vi "Strongrid_Core_app.vi"() -> ()   [LabVIEW 2013]
uses:
  Dependencies/Freq_select.ctl
  Dependencies/FrequencyKnob.ctl
  <vilib>/lvdsc/process/Undeploy Library.vi
  <vilib>/lvdsc/process/Deploy Library.vi
  <vilib>/S3DK/PMU Recorder Light/PMU Recorder Light.lvlib
  <vilib>/lvdsc/NI_DSC.lvlib
panel:
  in  "Ipad ON":bool
  in  "Ipad Display":bool
  out "low":bool caption="Low Frequency Warning"
  out "high":bool caption="High Frequency Warning"
  out "Xtra low":bool caption="Low Frequency Alarm"
  out "Xtra high":bool caption="High Frequency Alarm"
  out "TAMPERE":bool
  out "Aalto":bool
  out "Aalto Voltage":sgl
  out "Aalto Freq":T1 scale=49.85..50.15
  in  "V_select":T2 caption="Voltage Selection"
  out "Lund Frequency":T1 scale=49.85..50.15
  in  "Open PRL":bool
  out "Phasors":picture
  out "Buffer Active":bool
  out "Configuration File Received":bool
  out "Connected":bool
  out "Status Loop":bool
  out "Error":bool
  out "KTH Voltage":sgl
  out "KTH Frequency":T1 scale=49.85..50.15
  out "Chalmers Voltage":sgl
  out "Lund Voltage":sgl
  out "Tampere Voltage":sgl
  out "NTNU Voltage":sgl
  out "Tampere Frequency":T1 scale=49.85..50.15
  out "Chalmers Frequency":T1 scale=49.85..50.15
  out "NTNU Frequency":T1 scale=49.85..50.15
  out "LTU Voltage":sgl
  out "LTU Freq":T1 scale=49.85..50.15
  out "Lund PMU":bool
  out "Chalmers PMU":bool
  out "KTH PMU":bool
  out "NTNU PMU":bool
  out "LTU PMU":bool
  out "Has New Data?":bool
  out "Timed Loop":bool
  in  "Get Full Buffer?":bool
  in  "f_select":T2 caption="Frequency Selection"
  in  "Refresh Rate":u32(ring)=200 items=["20 Hz"=50, "10 Hz"=100, "5 Hz"=200, "2 Hz"=500, "1 Hz"=1000, "Every 2 sec"=2000, "Every 5 sec"=5000, "Every 10 sec"=10000, "Every minute"=4294961760]
  out "Quitting":bool
  out "Execution Loop":bool
  in  "Quit":bool
  out "Event Loop":bool
  out "Frequency":waveform(sgl)[](graph)
  out "Voltage":waveform(sgl)[](graph)
  # "USAGE:  Press play. The VI will start the PRL itself and wait for the connection to be established.\n(you will still need to configure the PRL first. If the Simple Frequency Reader works, then this works)"
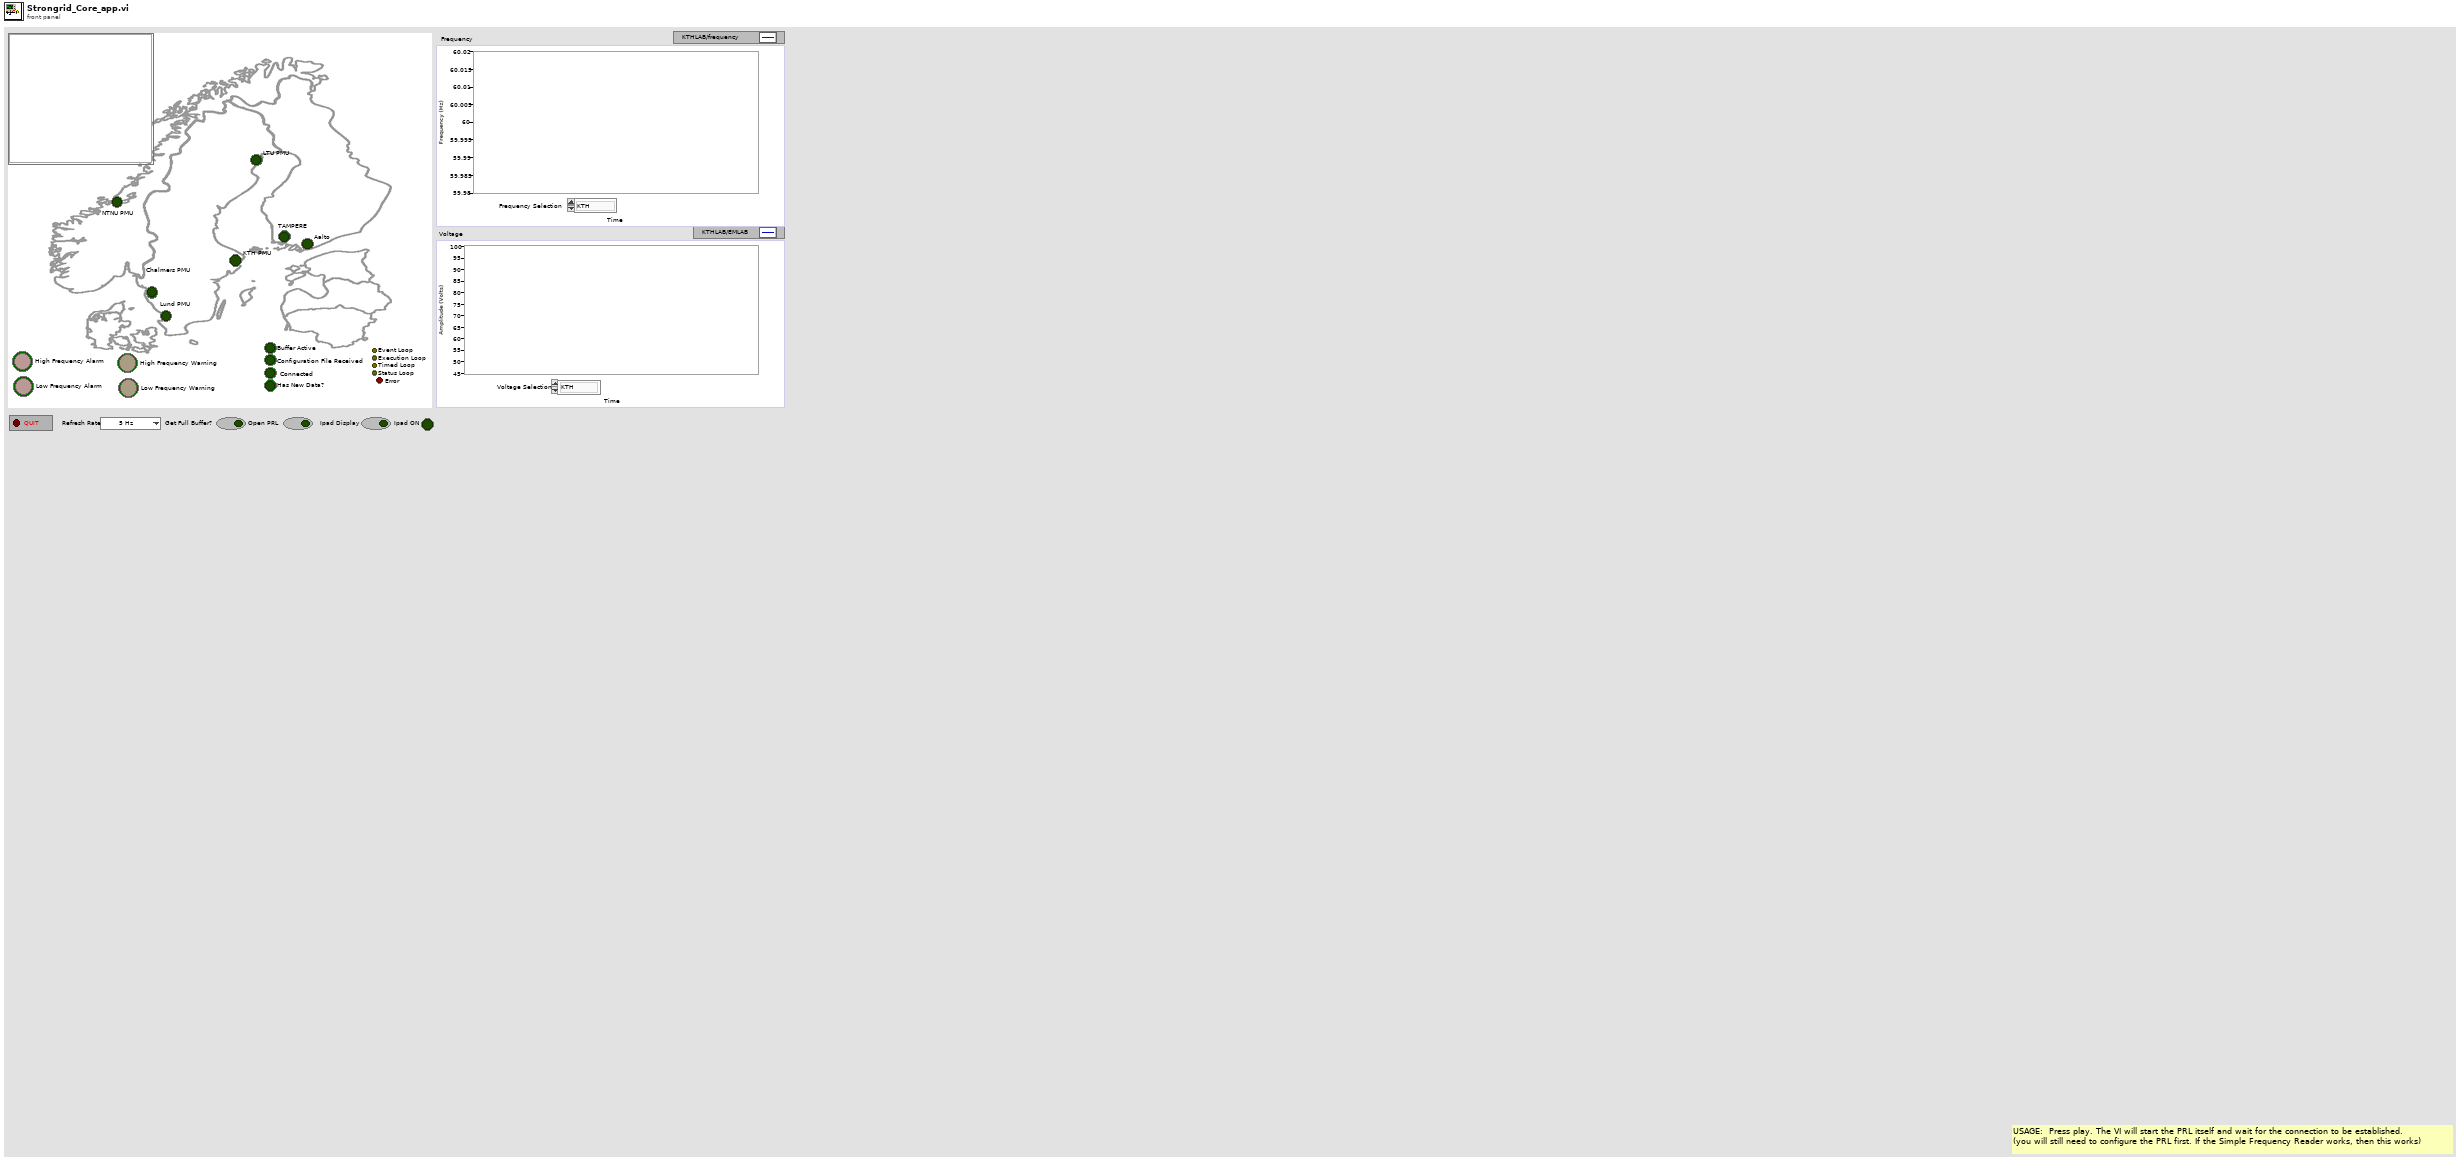
[diagram p1: front panel]
types:
  T1 = typedef "FrequencyKnob.ctl" = sgl
  T2 = typedef "Freq_select.ctl" = enum16{"KTH", "NTNU", "LTH", "CTH", "TAMPERE", "LTU", "Aalto", "ALL"}
  T3 = typedef "Semaphore RefNum" = refnum<k1>
  T4 = typedef "LVBoundsTypeDef.ctl" = cluster{"Width":u32, "Height":u32}
  T5 = enum16{"Run", "Startup", "Get Status", "Pause", "Continue", "Shutdown", "Abort", "Open Panel", "Close Panel"}
  T6 = cluster{"Phasor":string[], "Analog":string[], "Digital":string[]}
  T7 = enum16{"Filter Signals", "Get All Signal Names", "Select Signals on Name", "Select Frequency Only", "Get Selected Signal Names"}
  T8 = cluster{"KTH Voltage":refnum<vi>, "KTH Frequency":refnum<vi>}
  T9 = cluster{"LTU Voltage":refnum<vi>, "LTU Freq":refnum<vi>}
  T10 = cluster{"NTNU Voltage":refnum<vi>, "NTNU Frequency":refnum<vi>}
  T11 = cluster{"Chalmers Voltage":refnum<vi>, "Chalmers Frequency":refnum<vi>}
  T12 = cluster{"Lund Voltage":refnum<vi>, "Lund Frequency":refnum<vi>}
  T13 = cluster{"Tampere Voltage ":refnum<vi>, "Tampere Frequency":refnum<vi>}
  T14 = cluster{"Aalto Voltage":refnum<vi>, "Aalto Freq":refnum<vi>}
  T15 = cluster{"Analog Signals[0]":sgl, "Analog Signals[1]":sgl, "Analog Signals[2]":sgl, "Analog Signals[3]":sgl, "Analog Signals[4]":sgl, "Analog Signals[5]":sgl, "Analog Signals[6]":sgl}
  T16 = cluster{"[0]":sgl, "[1]":sgl, "[2]":sgl, "[3]":sgl, "[4]":sgl, "[5]":sgl, "[6]":sgl}
  T17 = cluster{"[0]":bool, "[1]":bool, "[2]":bool, "[3]":bool, "[4]":bool, "[5]":bool, "[6]":bool}
  T18 = cluster{"KTH":sgl, "NTNU":sgl, "Lund":sgl, "Chalmers":sgl, "Tampere":sgl, "LTU":sgl, "Aalto":sgl}
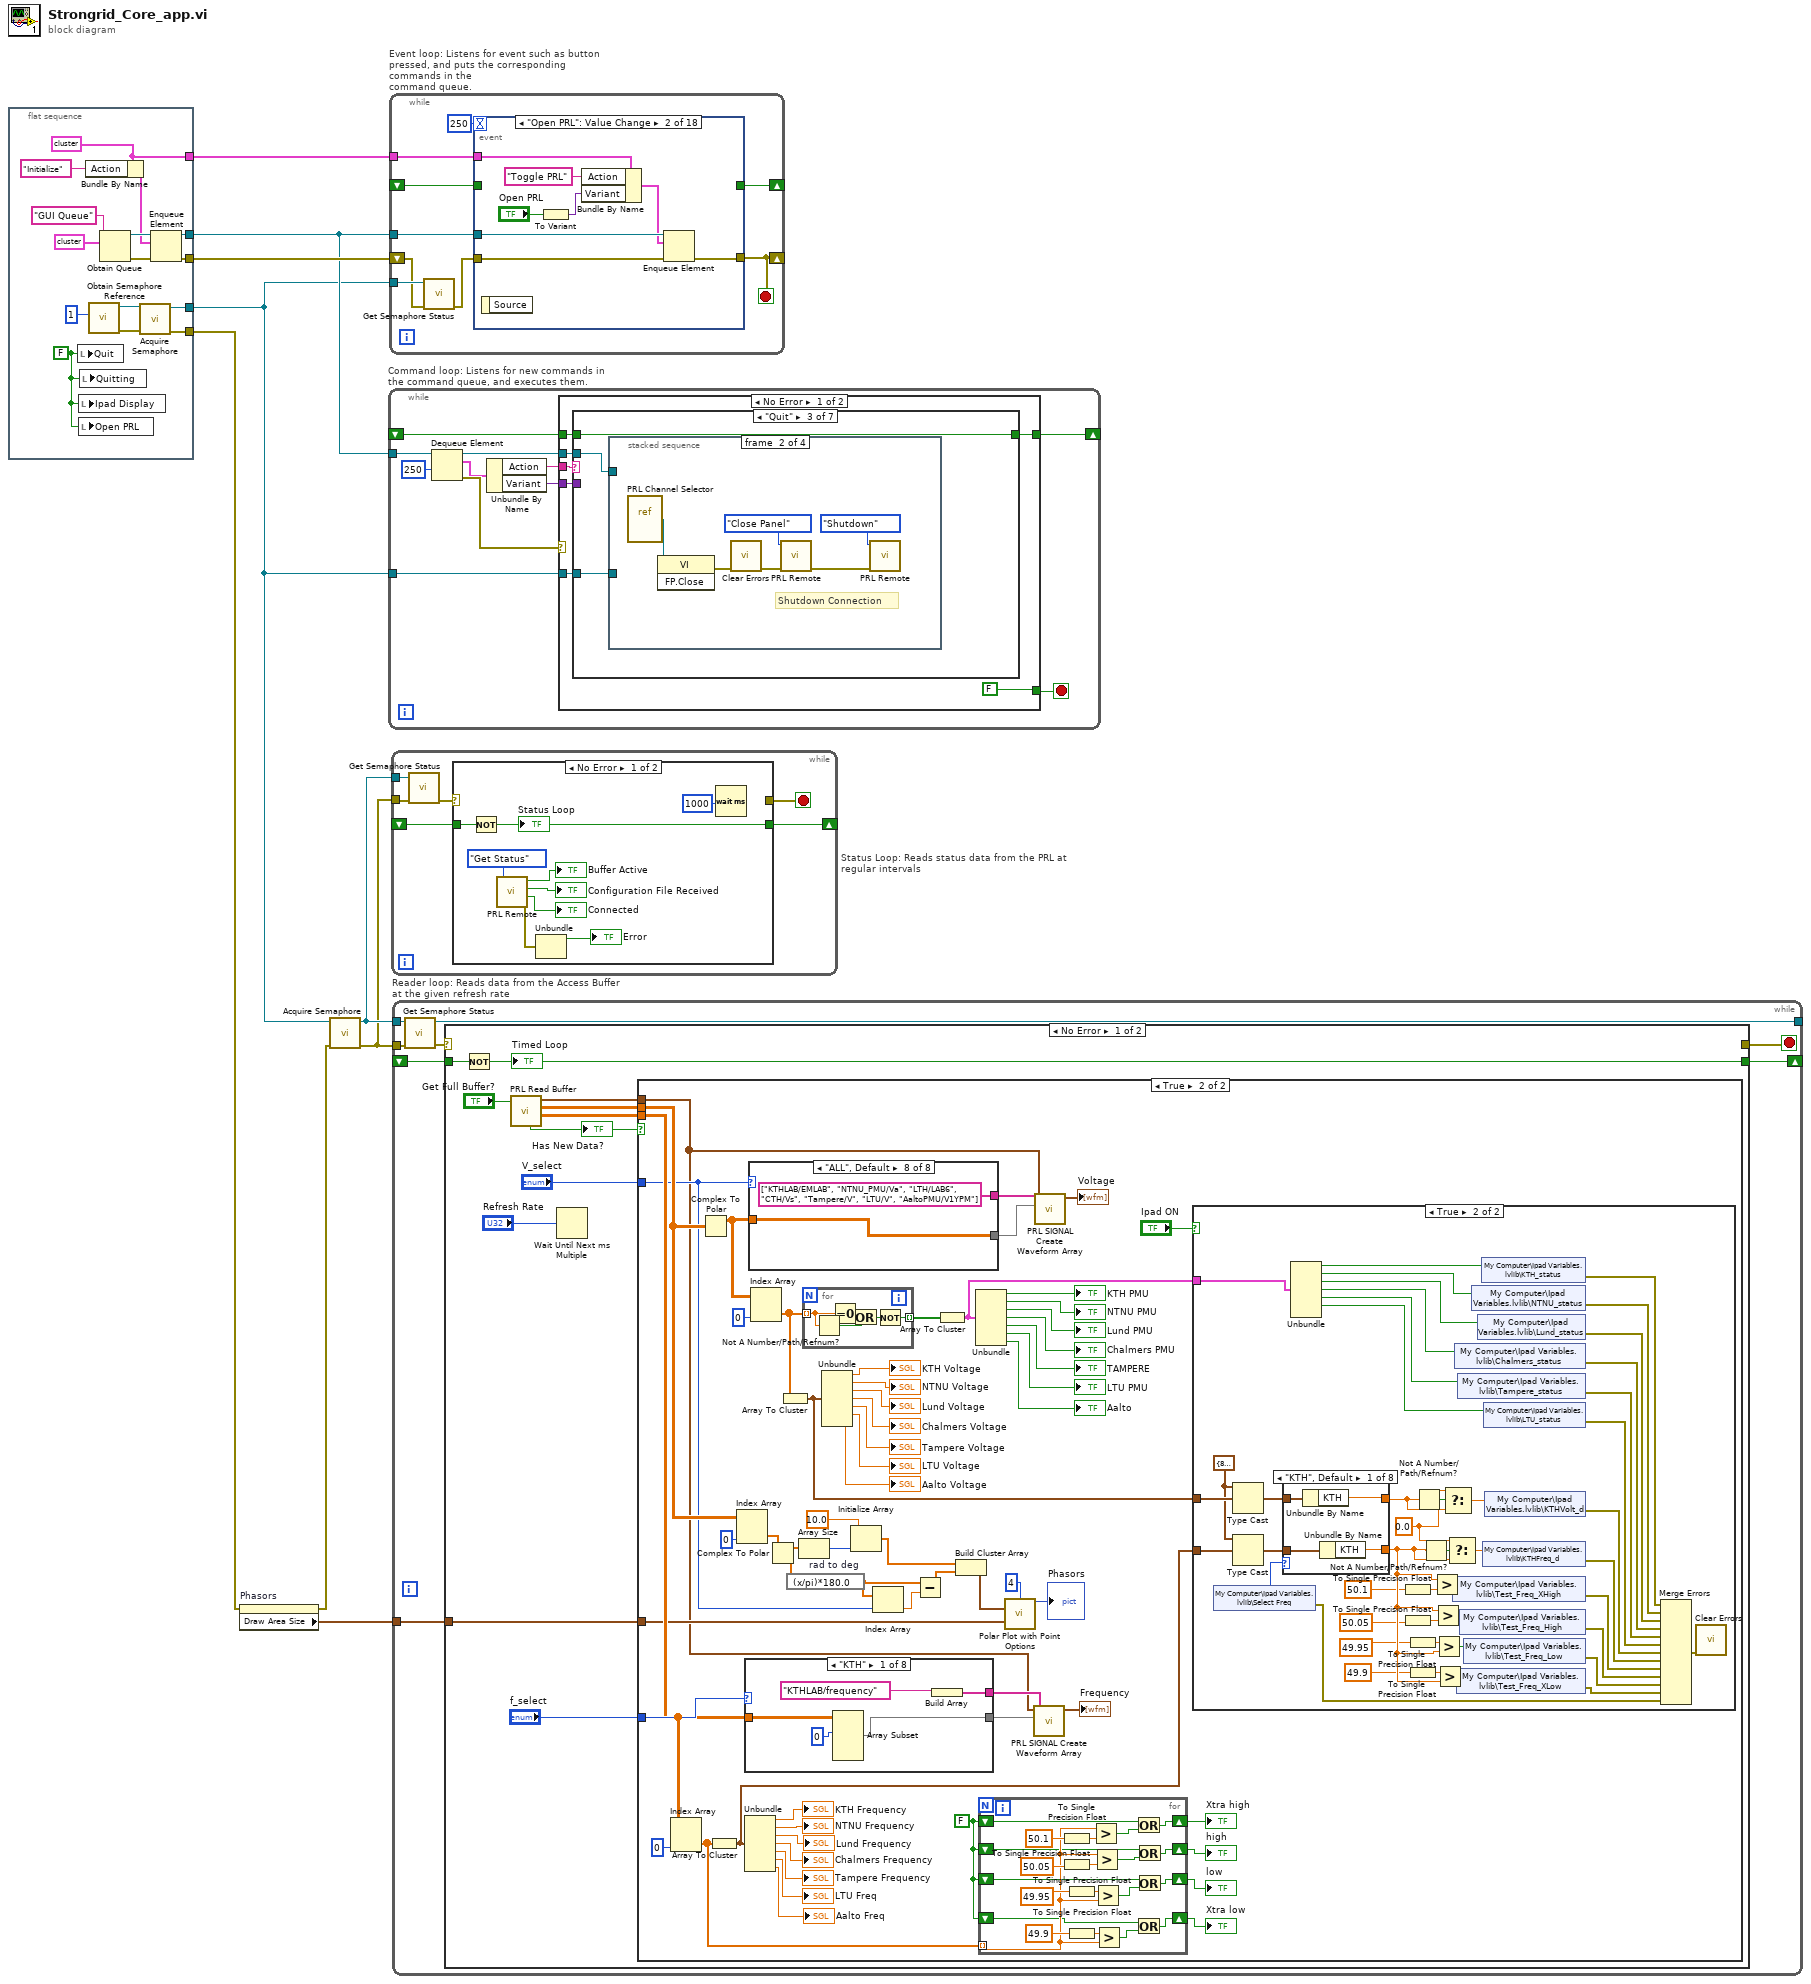
[diagram p0: block diagram]
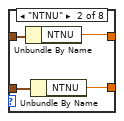
[diagram p5: hidden frame]
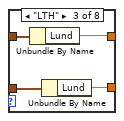
[diagram p6: hidden frame]
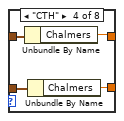
[diagram p7: hidden frame]
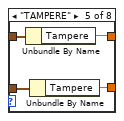
[diagram p8: hidden frame]
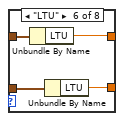
[diagram p9: hidden frame]
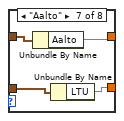
[diagram p10: hidden frame]
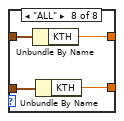
[diagram p11: hidden frame]
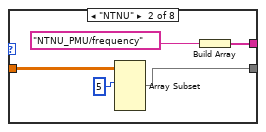
[diagram p12: hidden frame]
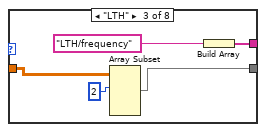
[diagram p13: hidden frame]
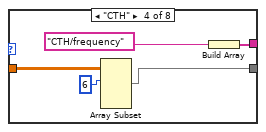
[diagram p14: hidden frame]
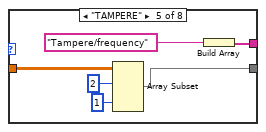
[diagram p15: hidden frame]
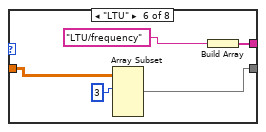
[diagram p16: hidden frame]
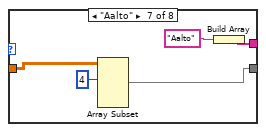
[diagram p17: hidden frame]
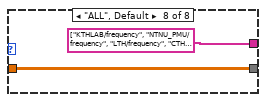
[diagram p18: hidden frame]
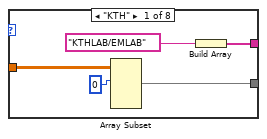
[diagram p19: hidden frame]
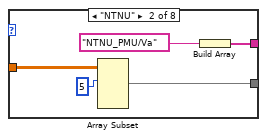
[diagram p20: hidden frame]
diagram:
  n1 = flat-sequence {
    tunnel: [w22] -> w9
    tunnel: [w21] -> w8
    tunnel: [w16] -> w7
    tunnel: [w12] -> w2
    tunnel: [w11] -> w1
    frame #0 {
      w10 = FALSE ("Quit")
      w16 = cluster{"Variant":variant, "Action":string} {"Variant"=variant, "Action"=""} ("Queue Element")
      n2 = local write "Quit"(w10) -> ()
      n3 = local write "Ipad Display"(w10) -> ()
      n4 = local write "Open PRL"(w10) -> ()
      n5 = local write "Quitting"(w10) -> ()
      n6 = Bundle By Name(cluster=w16, "Action"="Initialize" ("element")) -> (w17:cluster{"Variant":variant, "Action":string})
      n7 = call <vilib>:"Obtain Semaphore Reference.vi"("size (1)"=1) -> ("error out"=w15:errorcluster, "semaphore"=w14:T3)  [unwired: 4 in, 1 out]
      n8 = Obtain Queue(name (unnamed)="GUI Queue", element data type=cluster{"Variant":variant, "Action":string} {"Variant"=variant, "Action"=""} ("Queue Element")) -> (queue out=w24:refnum<queue>, error out=w23:errorcluster)  [unwired: 3 in, 1 out]
      n9 = call <vilib>:"Acquire Semaphore.vi"("error in (no error)"=w15, "semaphore"=w14) -> ("error out"=w12:errorcluster, "semaphore out"=w11:T3)  [unwired: 3 in, 1 out]
      n10 = Enqueue Element(queue=w24, element=w17, error in (no error)=w23) -> (queue out=w21:refnum<queue>, error out=w22:errorcluster)  [unwired: 1 in, 1 out]
    }
  }
  n11 = property on="Phasors" class="Pict"(error in=w2) -> (error out=w5:errorcluster, "Draw Area Size"=w6:T4)  [unwired: 1 in, 1 out]
  n12 = call <vilib>:"Acquire Semaphore.vi"("error in (no error)"=w5, "semaphore"=w1) -> ("error out"=w3:errorcluster, "semaphore out"=w4:T3)  [unwired: 3 in, 1 out]
  n13 = while "Command loop: Listens for new commands in the command queue, and executes them." {
    tunnel: w8 -> [w35]
    shift-right: [w30] -> _
    shift-left: _ -> [w31]
    tunnel: w1 -> [w25]
    stop <- w32 stop-if-true
    n14 = Dequeue Element(queue=w35, timeout in ms (-1)=250) -> (queue out=w33:refnum<queue>, element=w28:cluster{"Variant":variant, "Action":string}, error out=w34:errorcluster)  [unwired: 1 in, 1 out]
    n15 = Unbundle By Name(w28) -> ("Action"=w27:string, "Variant"=w26:variant)
    n16 = case shown="No Error" w34 {
      tunnel: w33 -> [w42 _]
      tunnel: [FALSE TRUE] -> w32
      tunnel: w31 -> [w40 w123]
      tunnel: [w39 w123] -> w30
      tunnel: w27 -> [w38 _]
      tunnel: w26 -> [w37 _]
      tunnel: w25 -> [w36 _]
      frame No Error {
        n17 = case shown="\"Quit\"" w38 {
          tunnel: w42 -> [_ _ w66 _ _ _ _]
          tunnel: w40 -> [w44 w46 w67 w80 w88 w96 w108]
          tunnel: [w43 w46 w67 w80 w88 w96 w108] -> w39
          tunnel: w37 -> [_ _ _ w84 w92 w101 w110]
          tunnel: w36 -> [_ w45 w65 _ _ _ _]
          frame "", Default {
            # "Switches the status indicator to \"Ready\",\nand alternates the Execution Loop indicator"
            n18 = Not(x=w44) -> (.not. x?=w43:bool)
            "Execution Loop" <- w43
          }
          frame "Initialize" {
            n19 = stacked-sequence {
              seq-local: [_ w50 _ _] -> [_ _ w60 _]
              tunnel: w45 -> [_ _ _ w64]
              frame #0 {
                # "Startup connection"
                # "Make sure quit\nis off"
                # "Run the PRL"
                n20 = call <vilib>:"PRL Remote.vi"("Action"=T5."Run") -> ("error out"=w47:errorcluster)  [unwired: 5 in, 5 out]
                n21 = call <vilib>:"PRL Remote.vi"("error in (no error)"=w47, "Action"=T5."Startup") -> ()  [unwired: 4 in, 6 out]
              }
              frame #1 {
                n22 = while {
                  tunnel: [w51] -> w50
                  i -> [w55]
                  stop <- w57 stop-if-true
                  # "Repeat until PRL is connected or quit is pressed"
                  n23 = Greater?(x=w55, y=10) -> (0:w53:bool)
                  n24 = local read "Quit"() -> (w52:bool)
                  n25 = Or(x=w52, y=w53) -> (x .or. y?=w51:bool)
                  n26 = call <vilib>:"PRL Remote.vi"("Action"=T5."Get Status") -> ("Connected"=w56:bool)  [unwired: 5 in, 5 out]
                  n27 = Or(x=w56, y=w51) -> (x .or. y?=w57:bool)
                  n28 = Wait (ms)(milliseconds to wait=u32 200) -> ()  [unwired: 1 out]
                }
              }
              frame #2 {
                n29 = case shown="False" w60 {
                  selector: w60 -> [_ w63]
                  frame False {
                    # "Select the frequency channels."
                    n30 = call <vilib>:"PRL Channel Selector Configuration.vi"("Signal Names In"=T6 {"Phasor"=["KTHLAB/EMLAB", "NTNU_PMU/Va", "LTH/LAB6", "CTH/Vs", "Tampere/V", "LTU/V", "AaltoPMU/V1YPM"], "Analog"=["KTHLAB/frequency", "NTNU_PMU/frequency", "LTH/frequency", "CTH/frequency", "Tampere/frequency", "LTU/frequency", "AaltoPMU/frequency"], "Digital"=[]}, "Action"=T7."Select Signals on Name") -> ()  [unwired: 9 in, 1 out]
                  }
                  frame True {
                    n31 = property on="Quit" class="Bool (strict)"("Val(Sgnl)"=w63) -> ()  [unwired: 2 in, 2 out]
                  }
                }
              }
              frame #3 {
                n32 = call <vilib>:"Release Semaphore.vi"("semaphore"=w64) -> ()  [unwired: 5 in, 2 out]
              }
            }
          }
          frame "Quit" {
            n33 = stacked-sequence {
              tunnel: w66 -> [_ _ w78 _]
              tunnel: w65 -> [_ _ w77 _]
              frame #0 {
                # "Indicator the Quitting sequence\nis engaged"
                "Quitting" <- TRUE ("Quitting")
              }
              frame #1 {
                # "Shutdown Connection"
                n34 = vi-ref <vilib>:"PRL Channel Selector.vi"() -> (w71:refnum<vi>)
                n35 = invoke class="VI" method="FP.Close"(reference=w71) -> (error out=w69:errorcluster)  [unwired: 2 in, 2 out]
                n36 = call <vilib>:"Clear Errors.vi"("error in (no error)"=w69) -> ("error out"=w70:errorcluster)  [unwired: 6 in]
                n37 = call <vilib>:"PRL Remote.vi"("error in (no error)"=w70, "Action"=T5."Close Panel") -> ("error out"=w72:errorcluster)  [unwired: 4 in, 5 out]
                n38 = call <vilib>:"PRL Remote.vi"("error in (no error)"=w72, "Action"=T5."Shutdown") -> ()  [unwired: 4 in, 6 out]
              }
              frame #2 {
                # "Removes the command queue\nwhich will cause this loop to\nend."
                n39 = Release Queue(queue=w78, force destroy? (F)=TRUE) -> ()  [unwired: 1 in, 3 out]
                n40 = call <vilib>:"Release Semaphore Reference.vi"("force destroy? (F)"=TRUE, "semaphore"=w77) -> ()  [unwired: 8 in, 2 out]
              }
              frame #3 {
                w79 = FALSE ("Quit")
                n41 = local write "Quit"(w79) -> ()
                n42 = local write "Ipad Display"(w79) -> ()
                n43 = local write "Quitting"(w79) -> ()
                n44 = local write "Open PRL"(w79) -> ()
              }
            }
          }
          frame "Enter" {
            # "Make Visible the correct indicators when overed by mouse"
            n45 = Variant To Data(type=T8 {"KTH Voltage"=refnum, "KTH Frequency"=refnum} ("output cluster"), Variant=w84) -> (data=w83:T8)  [unwired: 1 in, 1 out]
            n46 = Unbundle(w83) -> ("KTH Voltage"=w82:refnum<vi>, "KTH Frequency"=w81:refnum<vi>)
            n47 = property on="Property Node" class="DigNum (strict)"(reference=w82, "Visible"=TRUE) -> ()  [unwired: 1 in, 2 out]
            n48 = property on="Property Node" class="Knob (strict)"(reference=w81, "Visible"=TRUE) -> ()  [unwired: 1 in, 2 out]
          }
          frame "Leave" {
            # "Make invisible the correct indicators when mouse leaves"
            n49 = Variant To Data(type=T8 {"KTH Voltage"=refnum, "KTH Frequency"=refnum} ("output cluster"), Variant=w92) -> (data=w91:T8)  [unwired: 1 in, 1 out]
            n50 = Unbundle(w91) -> ("KTH Voltage"=w90:refnum<vi>, "KTH Frequency"=w89:refnum<vi>)
            n51 = property on="Property Node" class="DigNum (strict)"(reference=w90, "Visible"=FALSE) -> ()  [unwired: 1 in, 2 out]
            n52 = property on="Property Node" class="Knob (strict)"(reference=w89, "Visible"=FALSE) -> ()  [unwired: 1 in, 2 out]
          }
          frame "Toggle PRL" {
            n53 = Variant To Data(type=TRUE, Variant=w101) -> (data=w97:bool)  [unwired: 1 in, 1 out]
            n54 = Select(t=T5."Open Panel" ("Action"), s=w97, f=T5."Close Panel" ("Action")) -> (s? t:f=w100:T5)
            n55 = call <vilib>:"PRL Remote.vi"("Action"=w100) -> ()  [unwired: 5 in, 6 out]
          }
          frame "Toggle Ipad" {
            n56 = call <userlib>:"Current VI's Path (VI or exe).vi"() -> ("VI or executable installation directory"=w103:path)  [unwired: 14 in, 1 out]
            n57 = Variant To Data(type=TRUE, Variant=w110) -> (data=w109:bool)  [unwired: 1 in, 1 out]
            n58 = Build Path(base path=w103, name or relative path="Dependencies") -> (appended path=w106:path)
            n59 = Build Path(base path=w106, name or relative path="Ipad Variables.lvlib") -> (appended path=w104:path)
            n60 = case shown="True" w109 {
              tunnel: w104 -> [w112 w115]
              frame False {
                n61 = stacked-sequence {
                  tunnel: w112 -> [_ w114]
                  frame #0 {
                    n62 = local write "Ipad ON"(FALSE ("Ipad ON")) -> ()
                  }
                  frame #1 {
                    n63 = call-poly <vilib>:"Undeploy Libraries.vi"("library path"=w114) -> ()  [unwired: 8 in, 1 out]
                  }
                }
              }
              frame True {
                n64 = stacked-sequence {
                  tunnel: w115 -> [w116 _ _]
                  frame #0 {
                    n65 = call-poly <vilib>:"Deploy Libraries.vi"("library path"=w116) -> ()  [unwired: 8 in, 1 out]
                  }
                  frame #1 {
                    n66 = while {
                      stop <- w121 stop-if-true
                      n67 = shared-variable "My Computer\\Ipad Variables.lvlib\\Select Freq"(1000 ("ms timeout (0)")) -> (error out=w117:errorcluster, w120:bool)  [unwired: 1 in, 1 out]
                      n68 = shared-variable "My Computer\\Ipad Variables.lvlib\\Select Freq"(Freq_select."KTH" ("Select Freq"), error in=w117) -> ()  [unwired: 1 out]
                      n69 = Not(x=w120) -> (.not. x?=w121:bool)
                    }
                  }
                  frame #2 {
                    n70 = local write "Ipad ON"(TRUE ("Ipad ON")) -> ()
                  }
                }
              }
            }
          }
        }
      }
      frame Error {
      }
    }
  }
  n71 = while "Event loop: Listens for event such as button pressed, and puts the corresponding commands in the\ncommand queue." {
    shift-right: [w128] -> _
    shift-left: w9 -> [w126]
    tunnel: w8 -> [w133]
    shift-right: [w130] -> _
    shift-left: _ -> [w131]
    tunnel: w7 -> [w129]
    tunnel: w1 -> [w127]
    stop <- w128 stop-if-true
    n72 = call <vilib>:"Get Semaphore Status.vi"("error in (no error)"=w126, "semaphore"=w127) -> ("error out"=w125:errorcluster)  [unwired: 4 in, 5 out]
    n73 = event shown="[1] \"Open PRL\": Value Change" {
      selector: _ -> [_ _ _ _ _ _ _ _ _ _ _ _ _ _ _ _ _ _]
      dyn-events: _ -> [_ _ _ _ _ _ _ _ _ _ _ _ _ _ _ _ _ _]
      timeout: 250 -> [_ _ _ _ _ _ _ _ _ _ _ _ _ _ _ _ _ _]
      tunnel: w133 -> [_ w144 w152 w156 w174 w184 w194 w204 w214 w224 w234 w244 w254 w264 w274 w284 w294 w304]
      tunnel: w125 -> [w134 w138 w147 w157 w173 w183 w193 w203 w213 w223 w233 w243 w253 w263 w273 w283 w293 w303]
      tunnel: [w134 w137 w146 w153 w166 w176 w186 w196 w206 w216 w226 w236 w246 w256 w266 w276 w286 w296] -> w128
      tunnel: w131 -> [w136 _ _ _ _ _ _ _ _ _ _ _ _ _ _ _ _ _]
      tunnel: [w135 _ _ _ _ _ _ _ _ _ _ _ _ _ _ _ _ _] -> w130
      tunnel: w129 -> [_ w143 w151 w158 w171 w181 w191 w201 w211 w221 w231 w241 w251 w261 w271 w281 w291 w301]
      event Timeout {
        n74 = event-data() -> ()  [unwired: 1 in, 1 out]
        n75 = Not(x=w136) -> (.not. x?=w135:bool)
        "Event Loop" <- w135
      }
      event "Open PRL": Value Change {
        n76 = event-data() -> ()  [unwired: 1 in, 1 out]
        n77 = To Variant(anything="Open PRL") -> (Variant=w139:variant)
        n78 = Bundle By Name(cluster=w143, "Action"="Toggle PRL", "Variant"=w139) -> (w141:cluster{"Variant":variant, "Action":string})
        n79 = Enqueue Element(queue=w144, element=w141, error in (no error)=w138) -> (error out=w137:errorcluster)  [unwired: 1 in, 2 out]
      }
      event "Ipad Display": Value Change {
        n80 = event-data() -> ()  [unwired: 1 in, 1 out]
        n81 = To Variant(anything="Ipad Display") -> (Variant=w148:variant)
        n82 = Bundle By Name(cluster=w151, "Action"="Toggle Ipad", "Variant"=w148) -> (w149:cluster{"Variant":variant, "Action":string})
        n83 = Enqueue Element(queue=w152, element=w149, error in (no error)=w147) -> (error out=w146:errorcluster)  [unwired: 1 in, 2 out]
      }
      event "Quit": Value Change {
        n84 = event-data() -> ()  [unwired: 1 in, 1 out]
        n85 = To Variant(anything=FALSE ("Quit")) -> (Variant=w161:variant)
        n86 = Bundle By Name(cluster=w158, "Action"="Toggle Ipad", "Variant"=w161) -> (w159:cluster{"Variant":variant, "Action":string})
        n87 = Enqueue Element At Opposite End(queue=w156, element=w159, error in (no error)=w157) -> (queue out=w155:refnum<queue>, error out=w154:errorcluster)  [unwired: 1 in, 1 out]
        n88 = Bundle By Name(cluster=w158, "Action"="Quit" ("element")) -> (w163:cluster{"Variant":variant, "Action":string})
        n89 = Enqueue Element At Opposite End(queue=w155, element=w163, error in (no error)=w154) -> (error out=w153:errorcluster)  [unwired: 1 in, 2 out]
      }
      event "KTH PMU": Mouse Enter {
        n90 = event-data() -> ()  [unwired: 1 in, 1 out]
        n91 = control-ref of="KTH Frequency"() -> (w170:refnum<vi>)
        n92 = control-ref of="KTH Voltage"() -> (w169:refnum<vi>)
        n93 = Bundle("KTH Voltage"=w169, "KTH Frequency"=w170) -> (w167:T8)  [unwired: 1 in]
        n94 = To Variant(anything=w167) -> (Variant=w168:variant)
        n95 = Bundle By Name(cluster=w171, "Action"="Enter" ("element"), "Variant"=w168) -> (w165:cluster{"Variant":variant, "Action":string})
        n96 = Enqueue Element(queue=w174, element=w165, error in (no error)=w173) -> (error out=w166:errorcluster)  [unwired: 1 in, 2 out]
      }
      event "KTH PMU": Mouse Leave {
        n97 = event-data() -> ()  [unwired: 1 in, 1 out]
        n98 = control-ref of="KTH Frequency"() -> (w180:refnum<vi>)
        n99 = control-ref of="KTH Voltage"() -> (w179:refnum<vi>)
        n100 = Bundle("KTH Voltage"=w179, "KTH Frequency"=w180) -> (w177:T8)  [unwired: 1 in]
        n101 = To Variant(anything=w177) -> (Variant=w178:variant)
        n102 = Bundle By Name(cluster=w181, "Action"="Leave" ("element"), "Variant"=w178) -> (w175:cluster{"Variant":variant, "Action":string})
        n103 = Enqueue Element(queue=w184, element=w175, error in (no error)=w183) -> (error out=w176:errorcluster)  [unwired: 1 in, 2 out]
      }
      event "LTU PMU": Mouse Enter {
        n104 = event-data() -> ()  [unwired: 1 in, 1 out]
        n105 = control-ref of="LTU Freq"() -> (w190:refnum<vi>)
        n106 = control-ref of="LTU Voltage"() -> (w189:refnum<vi>)
        n107 = Bundle("LTU Voltage"=w189, "LTU Freq"=w190) -> (w187:T9)  [unwired: 1 in]
        n108 = To Variant(anything=w187) -> (Variant=w188:variant)
        n109 = Bundle By Name(cluster=w191, "Action"="Enter" ("element"), "Variant"=w188) -> (w185:cluster{"Variant":variant, "Action":string})
        n110 = Enqueue Element(queue=w194, element=w185, error in (no error)=w193) -> (error out=w186:errorcluster)  [unwired: 1 in, 2 out]
      }
      event "LTU PMU": Mouse Leave {
        n111 = event-data() -> ()  [unwired: 1 in, 1 out]
        n112 = control-ref of="LTU Freq"() -> (w200:refnum<vi>)
        n113 = control-ref of="LTU Voltage"() -> (w199:refnum<vi>)
        n114 = Bundle("LTU Voltage"=w199, "LTU Freq"=w200) -> (w197:T9)  [unwired: 1 in]
        n115 = To Variant(anything=w197) -> (Variant=w198:variant)
        n116 = Bundle By Name(cluster=w201, "Action"="Leave" ("element"), "Variant"=w198) -> (w195:cluster{"Variant":variant, "Action":string})
        n117 = Enqueue Element(queue=w204, element=w195, error in (no error)=w203) -> (error out=w196:errorcluster)  [unwired: 1 in, 2 out]
      }
      event "NTNU PMU": Mouse Enter {
        n118 = event-data() -> ()  [unwired: 1 in, 1 out]
        n119 = control-ref of="NTNU Frequency"() -> (w210:refnum<vi>)
        n120 = control-ref of="NTNU Voltage"() -> (w209:refnum<vi>)
        n121 = Bundle("NTNU Voltage"=w209, "NTNU Frequency"=w210) -> (w207:T10)  [unwired: 1 in]
        n122 = To Variant(anything=w207) -> (Variant=w208:variant)
        n123 = Bundle By Name(cluster=w211, "Action"="Enter" ("element"), "Variant"=w208) -> (w205:cluster{"Variant":variant, "Action":string})
        n124 = Enqueue Element(queue=w214, element=w205, error in (no error)=w213) -> (error out=w206:errorcluster)  [unwired: 1 in, 2 out]
      }
      event "NTNU PMU": Mouse Leave {
        n125 = event-data() -> ()  [unwired: 1 in, 1 out]
        n126 = control-ref of="NTNU Frequency"() -> (w220:refnum<vi>)
        n127 = control-ref of="NTNU Voltage"() -> (w219:refnum<vi>)
        n128 = Bundle("NTNU Voltage"=w219, "NTNU Frequency"=w220) -> (w217:T10)  [unwired: 1 in]
        n129 = To Variant(anything=w217) -> (Variant=w218:variant)
        n130 = Bundle By Name(cluster=w221, "Action"="Leave" ("element"), "Variant"=w218) -> (w215:cluster{"Variant":variant, "Action":string})
        n131 = Enqueue Element(queue=w224, element=w215, error in (no error)=w223) -> (error out=w216:errorcluster)  [unwired: 1 in, 2 out]
      }
      event "Chalmers PMU": Mouse Enter {
        n132 = event-data() -> ()  [unwired: 1 in, 1 out]
        n133 = control-ref of="Chalmers Frequency"() -> (w230:refnum<vi>)
        n134 = control-ref of="Chalmers Voltage"() -> (w229:refnum<vi>)
        n135 = Bundle("Chalmers Voltage"=w229, "Chalmers Frequency"=w230) -> (w227:T11)  [unwired: 1 in]
        n136 = To Variant(anything=w227) -> (Variant=w228:variant)
        n137 = Bundle By Name(cluster=w231, "Action"="Enter" ("element"), "Variant"=w228) -> (w225:cluster{"Variant":variant, "Action":string})
        n138 = Enqueue Element(queue=w234, element=w225, error in (no error)=w233) -> (error out=w226:errorcluster)  [unwired: 1 in, 2 out]
      }
      event "Chalmers PMU": Mouse Leave {
        n139 = event-data() -> ()  [unwired: 1 in, 1 out]
        n140 = control-ref of="Chalmers Frequency"() -> (w240:refnum<vi>)
        n141 = control-ref of="Chalmers Voltage"() -> (w239:refnum<vi>)
        n142 = Bundle("Chalmers Voltage"=w239, "Chalmers Frequency"=w240) -> (w237:T11)  [unwired: 1 in]
        n143 = To Variant(anything=w237) -> (Variant=w238:variant)
        n144 = Bundle By Name(cluster=w241, "Action"="Leave" ("element"), "Variant"=w238) -> (w235:cluster{"Variant":variant, "Action":string})
        n145 = Enqueue Element(queue=w244, element=w235, error in (no error)=w243) -> (error out=w236:errorcluster)  [unwired: 1 in, 2 out]
      }
      event "Lund PMU": Mouse Enter {
        n146 = event-data() -> ()  [unwired: 1 in, 1 out]
        n147 = control-ref of="Lund Frequency"() -> (w250:refnum<vi>)
        n148 = control-ref of="Lund Voltage"() -> (w249:refnum<vi>)
        n149 = Bundle("Lund Voltage"=w249, "Lund Frequency"=w250) -> (w247:T12)  [unwired: 1 in]
        n150 = To Variant(anything=w247) -> (Variant=w248:variant)
        n151 = Bundle By Name(cluster=w251, "Action"="Enter" ("element"), "Variant"=w248) -> (w245:cluster{"Variant":variant, "Action":string})
        n152 = Enqueue Element(queue=w254, element=w245, error in (no error)=w253) -> (error out=w246:errorcluster)  [unwired: 1 in, 2 out]
      }
      event "Lund PMU": Mouse Leave {
        n153 = event-data() -> ()  [unwired: 1 in, 1 out]
        n154 = control-ref of="Lund Frequency"() -> (w260:refnum<vi>)
        n155 = control-ref of="Lund Voltage"() -> (w259:refnum<vi>)
        n156 = Bundle("Lund Voltage"=w259, "Lund Frequency"=w260) -> (w257:T12)  [unwired: 1 in]
        n157 = To Variant(anything=w257) -> (Variant=w258:variant)
        n158 = Bundle By Name(cluster=w261, "Action"="Leave" ("element"), "Variant"=w258) -> (w255:cluster{"Variant":variant, "Action":string})
        n159 = Enqueue Element(queue=w264, element=w255, error in (no error)=w263) -> (error out=w256:errorcluster)  [unwired: 1 in, 2 out]
      }
      event "TAMPERE": Mouse Enter {
        n160 = event-data() -> ()  [unwired: 1 in, 1 out]
        n161 = control-ref of="Tampere Frequency"() -> (w270:refnum<vi>)
        n162 = control-ref of="Tampere Voltage"() -> (w269:refnum<vi>)
        n163 = Bundle("Tampere Voltage"=w269, "Tampere Frequency"=w270) -> (w267:T13)  [unwired: 1 in]
        n164 = To Variant(anything=w267) -> (Variant=w268:variant)
        n165 = Bundle By Name(cluster=w271, "Action"="Enter" ("element"), "Variant"=w268) -> (w265:cluster{"Variant":variant, "Action":string})
        n166 = Enqueue Element(queue=w274, element=w265, error in (no error)=w273) -> (error out=w266:errorcluster)  [unwired: 1 in, 2 out]
      }
      event "TAMPERE": Mouse Leave {
        n167 = event-data() -> ()  [unwired: 1 in, 1 out]
        n168 = control-ref of="Tampere Frequency"() -> (w280:refnum<vi>)
        n169 = control-ref of="Tampere Voltage"() -> (w279:refnum<vi>)
        n170 = Bundle("Tampere Voltage"=w279, "Tampere Frequency"=w280) -> (w277:T13)  [unwired: 1 in]
        n171 = To Variant(anything=w277) -> (Variant=w278:variant)
        n172 = Bundle By Name(cluster=w281, "Action"="Leave" ("element"), "Variant"=w278) -> (w275:cluster{"Variant":variant, "Action":string})
        n173 = Enqueue Element(queue=w284, element=w275, error in (no error)=w283) -> (error out=w276:errorcluster)  [unwired: 1 in, 2 out]
      }
      event "Aalto": Mouse Leave {
        n174 = event-data() -> ()  [unwired: 1 in, 1 out]
        n175 = control-ref of="Aalto Freq"() -> (w290:refnum<vi>)
        n176 = control-ref of="Aalto Voltage"() -> (w289:refnum<vi>)
        n177 = Bundle("Aalto Voltage"=w289, "Aalto Freq"=w290) -> (w287:T14)  [unwired: 1 in]
        n178 = To Variant(anything=w287) -> (Variant=w288:variant)
        n179 = Bundle By Name(cluster=w291, "Action"="Leave" ("element"), "Variant"=w288) -> (w285:cluster{"Variant":variant, "Action":string})
        n180 = Enqueue Element(queue=w294, element=w285, error in (no error)=w293) -> (error out=w286:errorcluster)  [unwired: 1 in, 2 out]
      }
      event "Aalto": Mouse Enter {
        n181 = event-data() -> ()  [unwired: 1 in, 1 out]
        n182 = control-ref of="Aalto Freq"() -> (w300:refnum<vi>)
        n183 = control-ref of="Aalto Voltage"() -> (w299:refnum<vi>)
        n184 = Bundle("Aalto Voltage"=w299, "Aalto Freq"=w300) -> (w297:T14)  [unwired: 1 in]
        n185 = To Variant(anything=w297) -> (Variant=w298:variant)
        n186 = Bundle By Name(cluster=w301, "Action"="Enter" ("element"), "Variant"=w298) -> (w295:cluster{"Variant":variant, "Action":string})
        n187 = Enqueue Element(queue=w304, element=w295, error in (no error)=w303) -> (error out=w296:errorcluster)  [unwired: 1 in, 2 out]
      }
    }
  }
  n188 = while "Status Loop: Reads status data from the PRL at regular intervals" {
    shift-right: [w309] -> _
    shift-left: _ -> [w310]
    tunnel: w4 -> [w308]
    tunnel: w3 -> [w307]
    stop <- w305 stop-if-true
    n189 = call <vilib>:"Get Semaphore Status.vi"("error in (no error)"=w307, "semaphore"=w308) -> ("error out"=w306:errorcluster)  [unwired: 4 in, 5 out]
    n190 = case shown="No Error" w306 {
      selector: w306 -> [_ w320]
      tunnel: w310 -> [w319 w321]
      tunnel: [w318 w321] -> w309
      tunnel: [_ w320] -> w305
      frame No Error {
        n191 = Not(x=w319) -> (.not. x?=w318:bool)
        "Status Loop" <- w318
        n192 = call <vilib>:"PRL Remote.vi"("Action"=T5."Get Status") -> ("error out"=w317:errorcluster, "Connected"=→"Connected":bool, "Configuration File Received"=→"Configuration File Received":bool, "Buffer Active"=→"Buffer Active":bool)  [unwired: 5 in, 2 out]
        n193 = Unbundle(w317) -> ("status"=→"Error":bool)  [unwired: 2 out]
        n194 = Wait (ms)(milliseconds to wait=u32 1000 ("Period")) -> ()  [unwired: 1 out]
      }
      frame Error {
      }
    }
  }
  n195 = while "Reader loop: Reads data from the Access Buffer at the given refresh rate" {
    tunnel: w3 -> [w326]
    tunnel: w4 -> [w325]
    shift-right: [w328] -> _
    shift-left: _ -> [w329]
    tunnel: w6 -> [w327]
    tunnel: [w324] -> _
    stop <- w322 stop-if-true
    n196 = call <vilib>:"Get Semaphore Status.vi"("error in (no error)"=w326, "semaphore"=w325) -> ("error out"=w323:errorcluster, "semaphore out"=w324:T3)  [unwired: 4 in, 4 out]
    n197 = case shown="No Error" w323 {
      selector: w323 -> [_ w582]
      tunnel: w329 -> [w333 w581]
      tunnel: [w332 w581] -> w328
      tunnel: w327 -> [w330 _]
      tunnel: [_ w582] -> w322
      frame No Error {
        n198 = Not(x=w333) -> (.not. x?=w332:bool)
        "Timed Loop" <- w332
        n199 = call <vilib>:"PRL Read Buffer .vi"("Get Full Buffer"="Get Full Buffer?") -> ("Analog Signals"=w339:sgl[][], "Phasor Signals"=w338:csg[][], "Timestamp"=w340:timestamp[], "Has Data"=w336:bool)  [unwired: 5 in, 2 out]
        "Has New Data?" <- w336
        n200 = Wait Until Next ms Multiple(millisecond multiple="Refresh Rate") -> ()  [unwired: 1 out]
        n201 = case shown="True" w336 {
          tunnel: w340 -> [_ w345]
          tunnel: w339 -> [_ w394]
          tunnel: w338 -> [_ w390]
          tunnel: "f_select" -> [_ w400]
          tunnel: "V_select" -> [_ w353]
          tunnel: w330 -> [_ w383]
          frame False {
          }
          frame True {
            w350 = FALSE
            n202 = Index Array(array=w394, index (col)=0 ("disabled index (col)")) -> (element=w351:sgl[])  [unwired: 1 in]
            n203 = Complex To Polar(r * e^(i*theta)=w390) -> (r=w352:sgl[][])  [unwired: 1 out]
            n204 = Array To Cluster(array=w351) -> (cluster=w343:T15)
            n205 = Index Array(array=w390, index (col)=0 ("disabled index (col)")) -> (element=w388:csg[])  [unwired: 1 in]
            n206 = case shown="\"KTH\"" w400 {
              tunnel: [w510 w515 w520 w525 w531 w536 w537 string[] ["KTHLAB/frequency", "NTNU_PMU/frequency", "LTH/frequency", "CTH/frequency", "Tampere/frequency", "LTU/frequency"] ("Analog")] -> w377
              tunnel: [w507 w511 w516 w521 w527 w532 w538 w542] -> w376
              tunnel: w394 -> [w506 w512 w517 w522 w528 w533 w539 w542]
              frame "KTH" {
                n207 = Array Subset(array=w506, index (row)=0 ("index")) -> (w507:sgl[][])  [unwired: 3 in]
                n208 = Build Array("KTHLAB/frequency" ("Station Name")) -> (w510:string[])
              }
              frame "NTNU" {
                n209 = Array Subset(array=w512, index (row)=5 ("index")) -> (w511:sgl[][])  [unwired: 3 in]
                n210 = Build Array("NTNU_PMU/frequency" ("Station Name")) -> (w515:string[])
              }
              frame "LTH" {
                n211 = Array Subset(array=w517, index (row)=2 ("index")) -> (w516:sgl[][])  [unwired: 3 in]
                n212 = Build Array("LTH/frequency" ("Station Name")) -> (w520:string[])
              }
              frame "CTH" {
                n213 = Array Subset(array=w522, index (row)=6 ("index")) -> (w521:sgl[][])  [unwired: 3 in]
                n214 = Build Array("CTH/frequency" ("Station Name")) -> (w525:string[])
              }
              frame "TAMPERE" {
                n215 = Array Subset(array=w528, index (row)=2 ("index"), length (row)=1 ("length")) -> (w527:sgl[][])  [unwired: 2 in]
                n216 = Build Array("Tampere/frequency" ("Station Name")) -> (w531:string[])
              }
              frame "LTU" {
                n217 = Array Subset(array=w533, index (row)=3 ("index")) -> (w532:sgl[][])  [unwired: 3 in]
                n218 = Build Array("LTU/frequency" ("Station Name")) -> (w536:string[])
              }
              frame "Aalto" {
                n219 = Array Subset(array=w539, index (row)=4 ("index")) -> (w538:sgl[][])  [unwired: 3 in]
                n220 = Build Array("Aalto" ("Station Name")) -> (w537:string[])
              }
              frame "ALL", Default {
              }
            }
            n221 = Unbundle(w343) -> ("Analog Signals[0]"=→"KTH Frequency":sgl, "Analog Signals[1]"=→"NTNU Frequency":sgl, "Analog Signals[2]"=→"Lund Frequency":sgl, "Analog Signals[3]"=→"Chalmers Frequency":sgl, "Analog Signals[4]"=→"Tampere Frequency":sgl, "Analog Signals[5]"=→"LTU Freq":sgl, "Analog Signals[6]"=→"Aalto Freq":sgl)
            n222 = case shown="\"ALL\", Default" w353 {
              tunnel: [w548 w553 w558 w563 w568 w573 w574 string[] ["KTHLAB/EMLAB", "NTNU_PMU/Va", "LTH/LAB6", "CTH/Vs", "Tampere/V", "LTU/V", "AaltoPMU/V1YPM"] ("Phasor")] -> w399
              tunnel: w352 -> [w545 w550 w555 w560 w565 w570 w576 w579]
              tunnel: [w546 w549 w554 w559 w564 w569 w575 w579] -> w393
              frame "KTH" {
                n223 = Array Subset(array=w545, index (row)=0 ("index")) -> (w546:sgl[][])  [unwired: 3 in]
                n224 = Build Array("KTHLAB/EMLAB" ("Station Name")) -> (w548:string[])
              }
              frame "NTNU" {
                n225 = Array Subset(array=w550, index (row)=5 ("index")) -> (w549:sgl[][])  [unwired: 3 in]
                n226 = Build Array("NTNU_PMU/Va" ("Station Name")) -> (w553:string[])
              }
              frame "LTH" {
                n227 = Array Subset(array=w555, index (row)=2 ("index")) -> (w554:sgl[][])  [unwired: 3 in]
                n228 = Build Array("LTH/LAB6" ("Station Name")) -> (w558:string[])
              }
              frame "CTH" {
                n229 = Array Subset(array=w560, index (row)=6 ("index")) -> (w559:sgl[][])  [unwired: 3 in]
                n230 = Build Array("CTH/Vs" ("Station Name")) -> (w563:string[])
              }
              frame "TAMPERE" {
                n231 = Array Subset(array=w565, index (row)=2 ("index")) -> (w564:sgl[][])  [unwired: 3 in]
                n232 = Build Array("Tampere/V" ("Station Name")) -> (w568:string[])
              }
              frame "LTU" {
                n233 = Array Subset(array=w570, index (row)=3 ("index")) -> (w569:sgl[][])  [unwired: 3 in]
                n234 = Build Array("LTU/V" ("Station Name")) -> (w573:string[])
              }
              frame "Aalto" {
                n235 = Array Subset(array=w576, index (row)=4 ("index")) -> (w575:sgl[][])  [unwired: 3 in]
                n236 = Build Array("Aalto" ("Station Name")) -> (w574:string[])
              }
              frame "ALL", Default {
              }
            }
            n237 = Index Array(array=w352, index (col)=0 ("disabled index (col)")) -> (element=w397:sgl[])  [unwired: 1 in]
            n238 = Complex To Polar(r * e^(i*theta)=w388) -> (r=w379:sgl[], theta=w391:sgl[])
            n239 = Array To Cluster(array=w397) -> (cluster=w344:T16)
            n240 = expression code="(x/pi)*180.0" "rad to deg"(w391) -> (w384:sgl[])
            n241 = Array Size(array=w379) -> (size(s)=w380:i32)
            n242 = for {
              tunnel: w397 -> [w502] mode=indexing
              tunnel: [w501] -> w396 mode=indexing
              n243 = Not A Number/Path/Refnum?(number/path/refnum=w502) -> (NaN/Path/Refnum?=w503:bool)
              n244 = Equal To 0?(x=w502) -> (x = 0?=w504:bool)
              n245 = Or(x=w504, y=w503) -> (x .or. y?=w505:bool)
              n246 = Not(x=w505) -> (.not. x?=w501:bool)
            }
            n247 = Unbundle(w344) -> ("[0]"=→"KTH Voltage":sgl, "[1]"=→"NTNU Voltage":sgl, "[2]"=→"Lund Voltage":sgl, "[3]"=→"Chalmers Voltage":sgl, "[4]"=→"Tampere Voltage":sgl, "[5]"=→"LTU Voltage":sgl, "[6]"=→"Aalto Voltage":sgl)
            n248 = Initialize Array(10.0 ("element"), w380) -> (w381:dbl[])
            n249 = Index Array(array=w384, index=w353) -> (element=w385:sgl)
            n250 = Subtract(x=w384, y=w385) -> (x-y=w386:sgl[])
            n251 = Array To Cluster(array=w396) -> (cluster=w342:T17)
            n252 = Build Cluster Array(w381, w386) -> (w387:cluster{"element":dbl, "element":sgl}[])
            n253 = Unbundle(w342) -> ("[0]"=→"KTH PMU":bool, "[1]"=→"NTNU PMU":bool, "[2]"=→"Lund PMU":bool, "[3]"=→"Chalmers PMU":bool, "[4]"=→"TAMPERE":bool, "[5]"=→"LTU PMU":bool, "[6]"=→"Aalto":bool)
            n254 = for {
              tunnel: w351 -> [w492] mode=indexing
              shift-right: [w482] -> w346
              shift-left: w350 -> [w480]
              shift-right: [w485] -> w347
              shift-left: w350 -> [w483]
              shift-right: [w488] -> w348
              shift-left: w350 -> [w486]
              shift-right: [w490] -> w349
              shift-left: w350 -> [w489]
              n255 = To Single Precision Float(number=50.1) -> (single precision float=w493:sgl)
              n256 = To Single Precision Float(number=50.05) -> (single precision float=w494:sgl)
              n257 = To Single Precision Float(number=49.95) -> (single precision float=w495:sgl)
              n258 = To Single Precision Float(number=49.9) -> (single precision float=w496:sgl)
              n259 = Greater?(x=w492, y=w493) -> (0:w491:bool)
              n260 = Greater?(x=w492, y=w494) -> (0:w487:bool)
              n261 = Greater?(x=w495, y=w492) -> (0:w484:bool)
              n262 = Greater?(x=w496, y=w492) -> (0:w481:bool)
              n263 = Or(x=w489, y=w491) -> (x .or. y?=w490:bool)
              n264 = Or(x=w480, y=w481) -> (x .or. y?=w482:bool)
              n265 = Or(x=w486, y=w487) -> (x .or. y?=w488:bool)
              n266 = Or(x=w483, y=w484) -> (x .or. y?=w485:bool)
            }
            "Xtra high" <- w349
            "Xtra low" <- w346
            "high" <- w348
            "low" <- w347
            n267 = call "Polar Plot with Point Options.vi"("data array [mag, phase (deg)]"=w387, "dimensions (w,h)"=w383, "Size"=u16 4) -> ("new picture"=→"Phasors":picture)  [unwired: 12 in]
            n268 = call <vilib>:"PRL SIGNAL Create Waveform Array.vi"("Signal Names"=w377, "Analog Signals"=w376, "Timestamp"=w345) -> ("Waveform Array"=→"Frequency":waveform(sgl)[])  [unwired: 8 in]
            n269 = call <vilib>:"PRL SIGNAL Create Waveform Array.vi"("Signal Names"=w399, "Analog Signals"=w393, "Timestamp"=w345) -> ("Waveform Array"=→"Voltage":waveform(sgl)[])  [unwired: 8 in]
            n270 = case shown="True" "Ipad ON" {
              tunnel: w344 -> [_ w447]
              tunnel: w343 -> [_ w446]
              tunnel: w342 -> [_ w445]
              frame False {
              }
              frame True {
                w444 = T18 {"KTH"=82.90574, "NTNU"=0.0, "Lund"=0.0, "Chalmers"=0.0, "Tampere"=0.0, "LTU"=0.0, "Aalto"=0.0} ("Cluster 2")
                w441 = sgl 0.0 ("element")
                n271 = shared-variable "My Computer\\Ipad Variables.lvlib\\Select Freq"() -> (w425:T2, error out=w414:errorcluster)  [unwired: 1 in]
                n272 = Type Cast(type=w444, x=w447) -> (*(type *) &x=w443:T18)
                n273 = Type Cast(type=w444, x=w446) -> (*(type *) &x=w442:T18)
                n274 = case shown="\"KTH\", Default" w425 {
                  tunnel: w442 -> [w451 w455 w459 w463 w467 w471 w474 w479]
                  tunnel: [w450 w454 w458 w462 w466 w470 w473 w478] -> w439
                  tunnel: w443 -> [w449 w453 w457 w461 w465 w469 w475 w477]
                  tunnel: [w448 w452 w456 w460 w464 w468 w472 w476] -> w440
                  frame "KTH", Default {
                    n275 = Unbundle By Name(w449) -> ("KTH"=w448:sgl)
                    n276 = Unbundle By Name(w451) -> ("KTH"=w450:sgl)
                  }
                  frame "NTNU" {
                    n277 = Unbundle By Name(w453) -> ("NTNU"=w452:sgl)
                    n278 = Unbundle By Name(w455) -> ("NTNU"=w454:sgl)
                  }
                  frame "LTH" {
                    n279 = Unbundle By Name(w457) -> ("Lund"=w456:sgl)
                    n280 = Unbundle By Name(w459) -> ("Lund"=w458:sgl)
                  }
                  frame "CTH" {
                    n281 = Unbundle By Name(w461) -> ("Chalmers"=w460:sgl)
                    n282 = Unbundle By Name(w463) -> ("Chalmers"=w462:sgl)
                  }
                  frame "TAMPERE" {
                    n283 = Unbundle By Name(w465) -> ("Tampere"=w464:sgl)
                    n284 = Unbundle By Name(w467) -> ("Tampere"=w466:sgl)
                  }
                  frame "LTU" {
                    n285 = Unbundle By Name(w469) -> ("LTU"=w468:sgl)
                    n286 = Unbundle By Name(w471) -> ("LTU"=w470:sgl)
                  }
                  frame "Aalto" {
                    n287 = Unbundle By Name(w475) -> ("Aalto"=w472:sgl)
                    n288 = Unbundle By Name(w474) -> ("LTU"=w473:sgl)
                  }
                  frame "ALL" {
                    n289 = Unbundle By Name(w477) -> ("KTH"=w476:sgl)
                    n290 = Unbundle By Name(w479) -> ("KTH"=w478:sgl)
                  }
                }
                n291 = Unbundle(w445) -> ("[0]"=w421:bool, "[1]"=w420:bool, "[2]"=w419:bool, "[3]"=w418:bool, "[4]"=w417:bool, "[5]"=w416:bool)  [unwired: 1 out]
                n292 = To Single Precision Float(number=50.1) -> (single precision float=w426:sgl)
                n293 = To Single Precision Float(number=50.05) -> (single precision float=w427:sgl)
                n294 = To Single Precision Float(number=49.95) -> (single precision float=w428:sgl)
                n295 = To Single Precision Float(number=49.9) -> (single precision float=w429:sgl)
                n296 = Not A Number/Path/Refnum?(number/path/refnum=w440) -> (NaN/Path/Refnum?=w438:bool)
                n297 = Not A Number/Path/Refnum?(number/path/refnum=w439) -> (NaN/Path/Refnum?=w437:bool)
                n298 = Greater?(x=w439, y=w426) -> (0:w435:bool)
                n299 = Greater?(x=w439, y=w427) -> (0:w424:bool)
                n300 = Greater?(x=w428, y=w439) -> (0:w423:bool)
                n301 = Greater?(x=w429, y=w439) -> (0:w422:bool)
                n302 = Select(t=w441, s=w438, f=w440) -> (s? t:f=w434:sgl)
                n303 = Select(t=w441, s=w437, f=w439) -> (s? t:f=w436:sgl)
                n304 = shared-variable "My Computer\\Ipad Variables.lvlib\\Test_Freq_XHigh"(w435) -> (error out=w411:errorcluster)  [unwired: 1 in]
                n305 = shared-variable "My Computer\\Ipad Variables.lvlib\\Chalmers_status"(w418) -> (error out=w406:errorcluster)  [unwired: 1 in]
                n306 = shared-variable "My Computer\\Ipad Variables.lvlib\\Test_Freq_XLow"(w422) -> (error out=w415:errorcluster)  [unwired: 1 in]
                n307 = shared-variable "My Computer\\Ipad Variables.lvlib\\Tampere_status"(w417) -> (error out=w407:errorcluster)  [unwired: 1 in]
                n308 = shared-variable "My Computer\\Ipad Variables.lvlib\\Test_Freq_High"(w424) -> (error out=w412:errorcluster)  [unwired: 1 in]
                n309 = shared-variable "My Computer\\Ipad Variables.lvlib\\Test_Freq_Low"(w423) -> (error out=w413:errorcluster)  [unwired: 1 in]
                n310 = shared-variable "My Computer\\Ipad Variables.lvlib\\NTNU_status"(w420) -> (error out=w404:errorcluster)  [unwired: 1 in]
                n311 = shared-variable "My Computer\\Ipad Variables.lvlib\\Lund_status"(w419) -> (error out=w405:errorcluster)  [unwired: 1 in]
                n312 = shared-variable "My Computer\\Ipad Variables.lvlib\\KTH_status"(w421) -> (error out=w403:errorcluster)  [unwired: 1 in]
                n313 = shared-variable "My Computer\\Ipad Variables.lvlib\\KTHFreq_d"(w436) -> (error out=w410:errorcluster)  [unwired: 1 in]
                n314 = shared-variable "My Computer\\Ipad Variables.lvlib\\LTU_status"(w416) -> (error out=w408:errorcluster)  [unwired: 1 in]
                n315 = shared-variable "My Computer\\Ipad Variables.lvlib\\KTHVolt_d"(w434) -> (error out=w409:errorcluster)  [unwired: 1 in]
                n316 = Merge Errors(w403, w404, w405, w406, w407, w408, w409, w410, w411, w412, w413, w415, w414) -> (w402:errorcluster)
                n317 = call <vilib>:"Clear Errors.vi"("error in (no error)"=w402) -> ()  [unwired: 6 in, 1 out]
              }
            }
          }
        }
      }
      frame Error {
      }
    }
  }
